vi "保存excel-电子表格.vi"(7 "测试数据":string[][](array[string]), 9 "保存路径":path, 10 "保存文件名称":string, 11 "标题":string) -> ()   [LabVIEW 2011]
uses:
  <vilib>/Utility/file.llb/Write To Spreadsheet File (string).vi
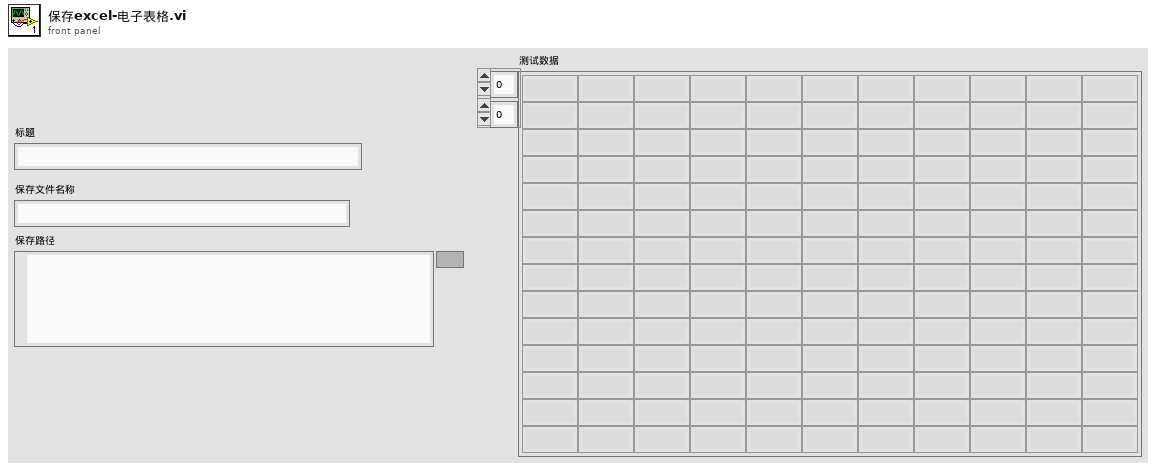
[diagram p1: front panel]
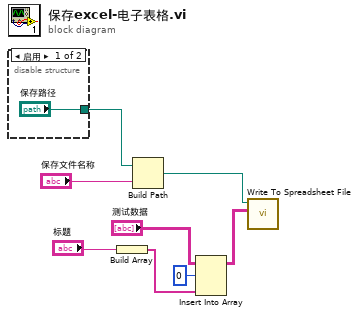
[diagram p0: block diagram]
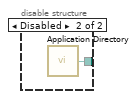
[diagram p2: hidden frame]
diagram:
  n1 = disable-structure shown="启用" {
    disable-tunnel: ["保存路径" w10] -> w7
    frame Enabled {
    }
    frame Disabled {
      n2 = call <vilib>:"Application Directory.vi"() -> ("Application Directory"=w10:path)
    }
  }
  n3 = Build Array("标题") -> (w3:string[])
  n4 = Build Path(base path=w7, name or relative path="保存文件名称") -> (appended path=w6:path)
  n5 = Insert Into Array(array="测试数据", index (row)=0 ("索引 (行)"), new element=w3) -> (w2:string[][])  [unwired: 1 in]
  n6 = call-poly <vilib>:"Write To Spreadsheet File.vi"("2D data"=w2, "file path (dialog if empty)"=w6) -> ()  [unwired: 6 in, 1 out]
